vi "Read Cabin.vi"(8 "error in (no error)":errorcluster, 11 "Change Inlet MSG in":refnum<class "Change Inlet MSG.lvclass">) -> (0 "error out":errorcluster, 2 "Cabin":bool, 3 "Change Inlet MSG out":refnum<class "Change Inlet MSG.lvclass">)   [LabVIEW 2014, in "Controller.lvlib" / "Change Inlet MSG.lvclass"]
uses:
  Change Inlet MSG.lvclass
  Change Inlet MSG.lvclass/Change Inlet MSG.ctl
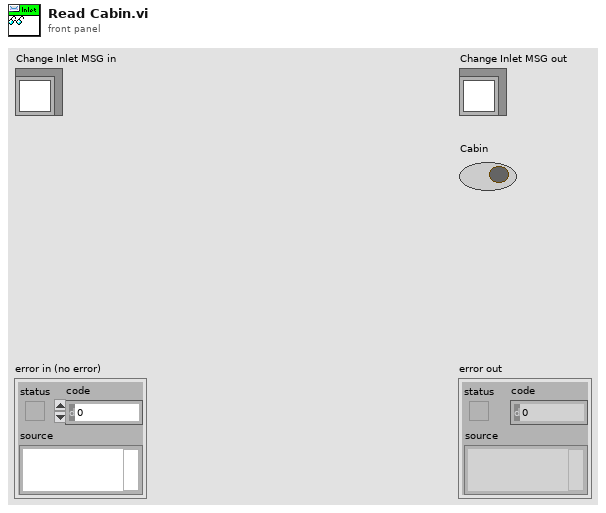
[diagram p1: front panel]
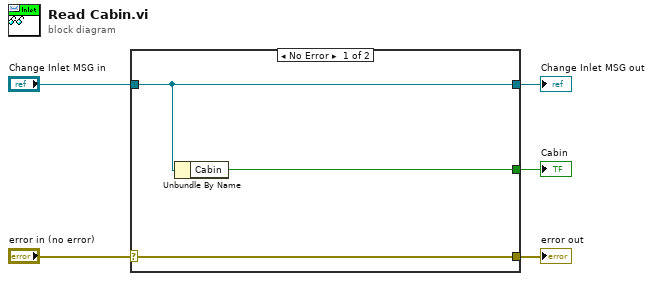
[diagram p0: block diagram]
diagram:
  n1 = case shown="No Error" "error in (no error)" {
    selector: "error in (no error)" -> [w8 w9]
    tunnel: [w8 w9] -> w4
    tunnel: [w7 w10] -> w2
    tunnel: "Change Inlet MSG in" -> [w7 w10]
    tunnel: [w6 _] -> w1
    frame No Error {
      n2 = Unbundle By Name(w7) -> ("Cabin"=w6:bool)
    }
    frame Error {
    }
  }
  "error out" <- w4
  "Change Inlet MSG out" <- w2
  "Cabin" <- w1
